vi "Check Car Position.vi"(8 "error in (no error)":errorcluster, 10 "Car Position Slider":u8(slide) max=3 scale=0.0..4.0, 11 "Car Wash Steps":string[][](array[string])) -> (0 "error out":errorcluster, 3 "Position Correct?":bool)   [LabVIEW 2020]
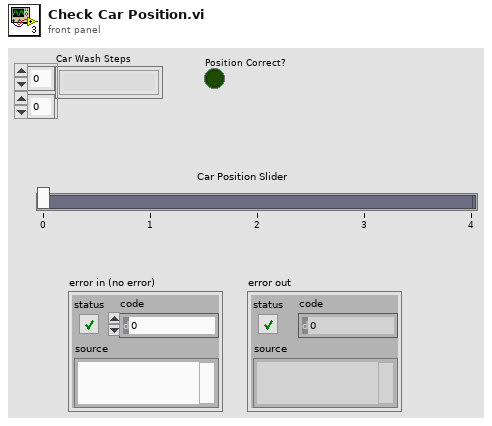
[diagram p1: front panel]
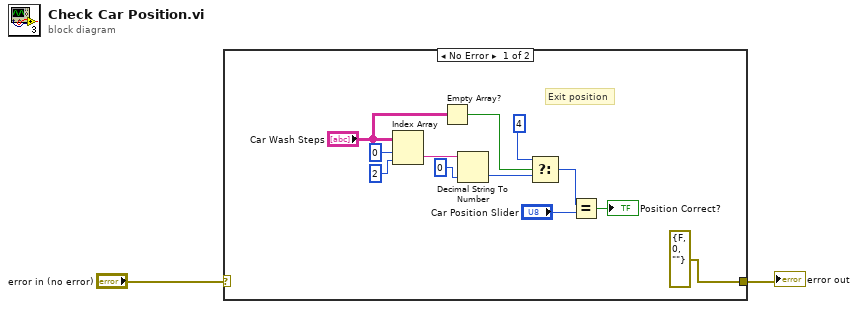
[diagram p0: block diagram]
diagram:
  n1 = case shown="No Error" "error in (no error)" {
    selector: "error in (no error)" -> [_ w15]
    tunnel: [errorcluster {"status"=FALSE, "code"=0, "source"=""} ("error IO") w15] -> w1
    frame No Error {
      # "Exit position"
      n2 = Index Array(array="Car Wash Steps", index (row)=0, index (col)=2 ("disabled index (col)")) -> (element=w12:string)
      n3 = Empty Array?(array="Car Wash Steps") -> (empty?=w6:bool)
      n4 = Decimal String To Number(string=w12, default (0L)=u8 0 ("default (0 I32)")) -> (number=w5:u8)  [unwired: 1 in, 1 out]
      n5 = Select(t=u8 4, s=w6, f=w5) -> (s? t:f=w3:u8)
      n6 = Equal?(x=w3, y="Car Position Slider") -> (x = y?=→"Position Correct?":bool)
    }
    frame Error {
    }
  }
  "error out" <- w1
